vi "KGN Set Limits.vi"(7 "Limits Cluster in":cluster{"flow":dbl[], "temp":dbl[]}, 8 "Fehler (Eingang, kein Fehler)":errorcluster, 9 "Info Cluster":T1, 10 "VISA-Referenz (Eingang)":refnum<visa-resource-name>, 11 "device (Eingang)":u32) -> (0 "Fehler (Ausgang)":errorcluster, 1 "Info Cluster out":T1, 2 "VISA-Referenz (Ausgang)":refnum<visa-resource-name>, 3 "dup device (Ausgang)":u32, 4 "Kommandos gesendet":string)   [LabVIEW 2020, in "Linearisierung v2.lvlib" / "Gasteiler.lvlib" / "HovaCAL_Interface.lvlib" / "KGN.lvlib" / "KGN GUI Set.lvlib"]
uses:
  KGN GUI Set.lvlib
  Controls/Info Cluster.ctl
  set/set.lvlib
  Controls/Controls.lvlib
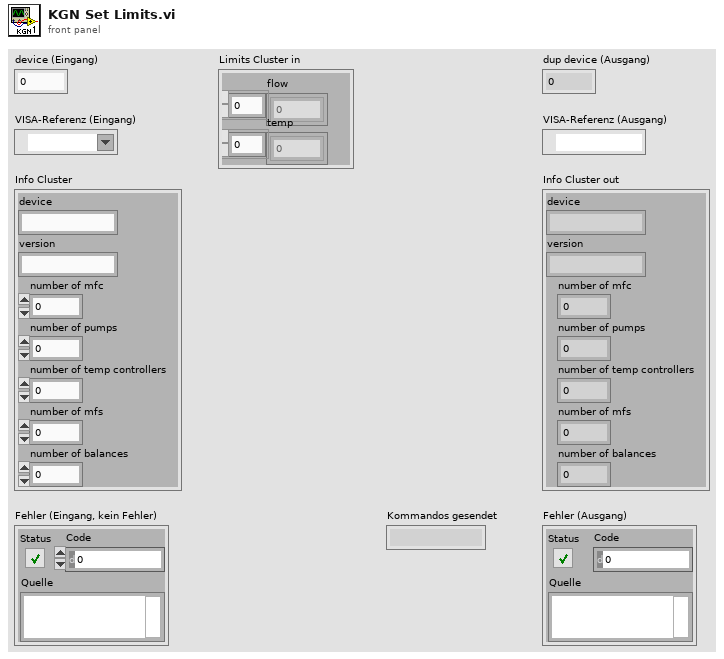
[diagram p1: front panel]
types:
  T1 = typedef "Linearisierung v2.lvlib/Gasteiler.lvlib/HovaCAL_Interface.lvlib/Controls.lvlib/Info Cluster.ctl" = cluster{"device":string, "version":string, "number of mfc":i32, "number of pumps":i32, "number of temp controllers":i32, "number of mfs":i32, "number of balances":i32}
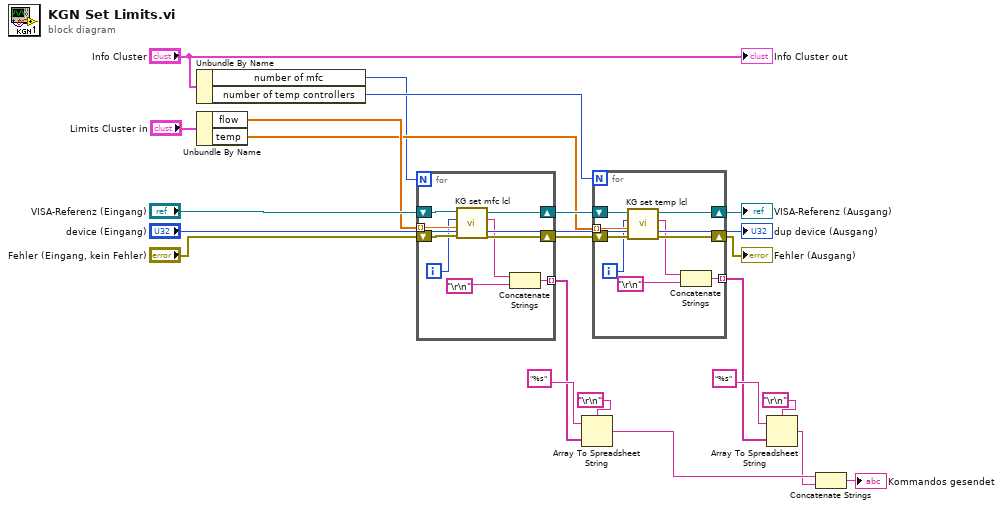
[diagram p0: block diagram]
diagram:
  n1 = Unbundle By Name("Info Cluster") -> ("number of mfc"=w10:i32, "number of temp controllers"=w11:i32)
  n2 = Unbundle By Name("Limits Cluster in") -> ("flow"=w13:dbl[], "temp"=w12:dbl[])
  n3 = for {
    N: w10 -> [_]
    tunnel: w13 -> [w27] mode=indexing
    shift-right: [w28] -> w17
    shift-left: "Fehler (Eingang, kein Fehler)" -> [w31]
    shift-right: [w29] -> w18
    shift-left: "VISA-Referenz (Eingang)" -> [w30]
    tunnel: [w23] -> w7 mode=indexing
    i -> [w26]
    n4 = call "KG set mfc lcl.vi"("Fehler (Eingang, kein Fehler)"=w31, "flow"=w27, "mfc"=w26, "VISA-Ressourcenname"=w30) -> ("Fehler (Ausgang)"=w28:errorcluster, "Kommando gesendet"=w24:string, "VISA-Ressourcenname (Ausgang)"=w29:refnum<visa-resource-name>)  [unwired: 5 in]
    n5 = Concatenate Strings(w24, "\r\n") -> (w23:string)
  }
  n6 = Array To Spreadsheet String(delimiter (Tab)="\r\n", array=w7, 3:"%s" ("Format-String")) -> (spreadsheet string=w4:string)
  n7 = for {
    N: w11 -> [_]
    tunnel: w12 -> [w36] mode=indexing
    shift-right: [w38] -> w16
    shift-left: w18 -> [w40]
    shift-right: [w37] -> w15
    shift-left: w17 -> [w39]
    tunnel: [w32] -> w5 mode=indexing
    i -> [w35]
    n8 = call "KG set temp lcl.vi"("Fehler (Eingang, kein Fehler)"=w39, "temp"=w36, "controller"=w35, "VISA-Ressourcenname"=w40) -> ("Fehler (Ausgang)"=w37:errorcluster, "Kommando gesendet"=w33:string, "VISA-Ressourcenname (Ausgang)"=w38:refnum<visa-resource-name>)  [unwired: 5 in]
    n9 = Concatenate Strings(w33, "\r\n") -> (w32:string)
  }
  "Fehler (Ausgang)" <- w15
  "VISA-Referenz (Ausgang)" <- w16
  n10 = Array To Spreadsheet String(delimiter (Tab)="\r\n", array=w5, 3:"%s" ("Format-String")) -> (spreadsheet string=w1:string)
  n11 = Concatenate Strings(w4, w1) -> (→"Kommandos gesendet":string)
  "dup device (Ausgang)" <- "device (Eingang)"
  "Info Cluster out" <- "Info Cluster"
